vi "Update Electric Test Only.vi"(8 "error in (no error)":errorcluster) -> (0 "error out":errorcluster, 3 "Electric Test Only status":bool)   [LabVIEW 2015]
uses:
  C:/C-BOX_DoIP/Utilities/dotNET/C-BOX_DoIP/INIFileParser.dll
  C-BOX_DoIP/Utilities/dotNET/C-BOX_DoIP/INIFileParser.dll
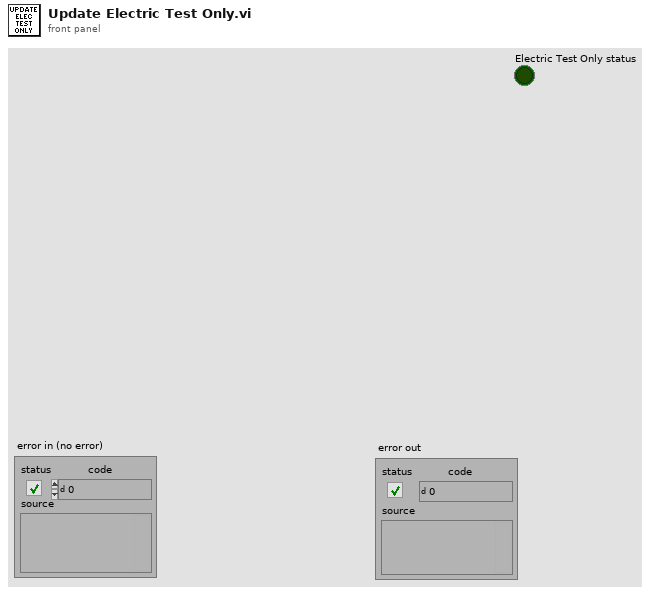
[diagram p1: front panel]
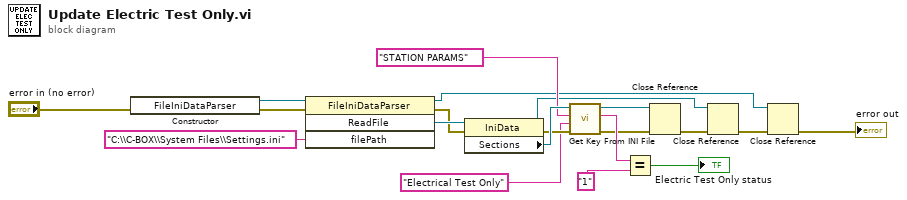
[diagram p0: block diagram]
diagram:
  n1 = constructor class="FileIniDataParser"(error in="error in (no error)") -> (reference out=w20:refnum<k24>, error out=w19:errorcluster)  [unwired: 2 in, 1 out]
  n2 = invoke class="FileIniDataParser" method="ReadFile"(reference=w20, error in=w19, "filePath"="C:\\C-BOX\\System Files\\Settings.ini") -> (reference out=w3:refnum<k24>, error out=w16:errorcluster, "ReadFile"=w17:refnum<k24>)  [unwired: 1 in, 1 out]
  n3 = property class="IniData"(reference=w17, error in=w16) -> (reference out=w5:refnum<k24>, error out=w14:errorcluster, "Sections"=w15:refnum<k24>)
  n4 = call "Get Key From INI File.vi"("error in (no error)"=w14, "keyName"="Electrical Test Only", "sectionName"="STATION PARAMS", "Sections in"=w15) -> ("error out"=w8:errorcluster, "keyValue"=w11:string, "Sections out"=w7:refnum<k24>)  [unwired: 5 in]
  n5 = Equal?(x=w11, y="1") -> (x = y?=→"Electric Test Only status":bool)
  n6 = Close Reference(reference=w7, error in (no error)=w8) -> (error out=w6:errorcluster)
  n7 = Close Reference(reference=w5, error in (no error)=w6) -> (error out=w4:errorcluster)
  n8 = Close Reference(reference=w3, error in (no error)=w4) -> (error out=→"error out":errorcluster)
